vi "FTW-Actor-Initialized.vi"(0 "FTW Actor Instance":refnum<class "FTW-Actor-Instance.lvclass">, 5 "Initialized Response":string, 11 "error in":errorcluster) -> (4 "FTW Actor Instance out":refnum<class "FTW-Actor-Instance.lvclass">, 6 "Timed out?":bool, 15 "error out":errorcluster)   [LabVIEW 2013, in "FTW-Actor-Instance.lvclass"]
uses:
  FTW-Actor-Instance.lvclass
  FTW-Actor-FrameworkEvent.ctl
  FTW-Actor-Instance.lvclass/FTW-Actor-Instance.ctl
  time/FTW-Time-DisplayFormat-Timestamp.ctl
  socket/FTW-Socket-Type.ctl
  socket/FTW-Socket.lvclass
panel:
  # "Inputs"
  # "Outputs"
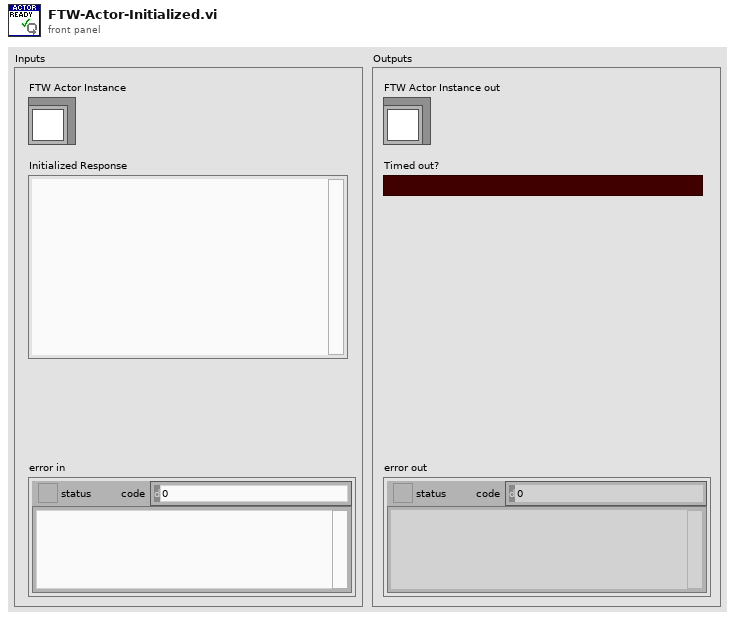
[diagram p1: front panel]
types:
  T1 = typedef "FTW-Actor-Instance.lvclass/FTW-Actor-FrameworkEvent.ctl" = enum16{"Instance Initializing", "Instance Initialized", "Instance Job", "Instance Handle Request", "Instance Shutting Down", "Instance Destroyed"}
  T2 = typedef "FTW-Time-DisplayFormat-Timestamp.ctl" = enum16{"YYYY-MM-DDT00:00:00.000Z (ISO-8601)", "YYYY-MM-DDT00-00-00Z (Simple ISO-8601)", "YYYY-MM-DD"}
  T3 = typedef "FTW-Socket.lvclass/FTW-Socket-Type.ctl" = enum32{"Server", "Client", "Publisher", "Subscriber", "Pipeline Producer", "Pipeline Consumer", "Surveyor", "Respondent", "Exclusive Pair", "Bus"}
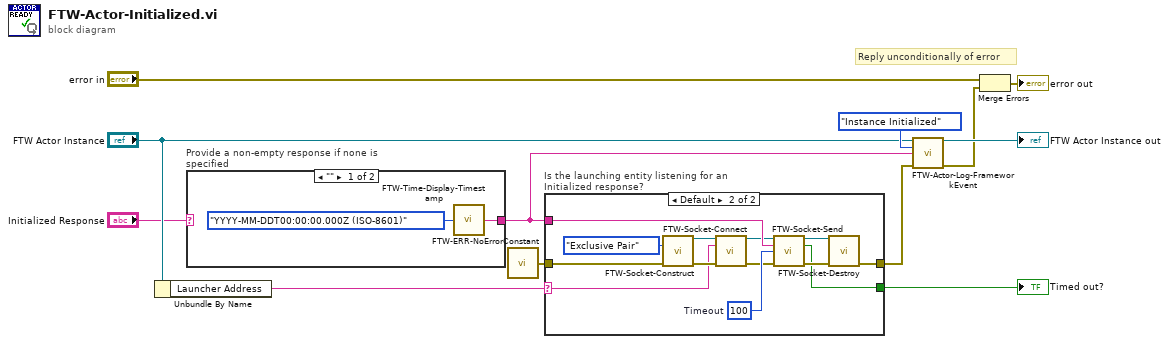
[diagram p0: block diagram]
diagram:
  # "Reply unconditionally of error"
  n1 = Unbundle By Name("FTW Actor Instance") -> ("Launcher Address"=w8:string)
  n2 = case "Provide a non-empty response if none is specified" shown="\"\"" "Initialized Response" {
    selector: "Initialized Response" -> [_ w15]
    tunnel: [w14 w15] -> w6
    frame "" {
      n3 = call "FTW-Time-Display-Timestamp.vi"("Format"=FTW-Time-DisplayFormat-Timestamp."YYYY-MM-DDT00:00:00.000Z (ISO-8601)") -> ("Formatted Timestamp"=w14:string)  [unwired: 3 in]
    }
    frame Default {
    }
  }
  n4 = call "FTW-ERR-NoErrorConstant.vi"() -> ("no error"=w5:errorcluster)
  n5 = case "Is the launching entity listening for an Initialized response?" shown="Default" w8 {
    selector: w8 -> [_ w21]
    tunnel: w6 -> [_ w28]
    tunnel: [w16 w26] -> w9
    tunnel: w5 -> [w16 w20]
    tunnel: [_ w18] -> w1
    frame "" {
    }
    frame Default {
      w25 = 100  # Timeout
      n6 = call "FTW-Socket-Construct.vi"("Socket Topology"=FTW-Socket-Type."Exclusive Pair" ("Socket Type"), "error in"=w20) -> ("FTW Socket"=w23:refnum<class "FTW-Socket.lvclass">, "error out"=w22:errorcluster)  [unwired: 12 in]
      n7 = call "FTW-Socket-Connect.vi"("FTW Socket"=w23, "Remote Address"=w21, "error in"=w22) -> ("FTW Socket out"=w19:refnum<class "FTW-Socket.lvclass">, "error out"=w17:errorcluster)  [unwired: 11 in]
      n8 = call "FTW-Socket-Send.vi"("FTW Socket"=w19, "Message"=w28, "Send Timeout"=w25, "error in"=w17) -> ("FTW Socket out"=w29:refnum<class "FTW-Socket.lvclass">, "Timed out?"=w18:bool, "error out"=w27:errorcluster)  [unwired: 9 in]
      n9 = call-dynamic "FTW-Socket-Destroy.vi"("FTW Socket"=w29, "error in"=w27) -> ("error out"=w26:errorcluster)  [unwired: 13 in]
    }
  }
  "Timed out?" <- w1
  n10 = call "FTW-Actor-Log-FrameworkEvent.vi"("FTW Actor Instance"="FTW Actor Instance", "Framework Event"=FTW-Actor-FrameworkEvent."Instance Initialized", "Event Data"=w6, "error in"=w9) -> ("FTW Actor Instance out"=→"FTW Actor Instance out":refnum<class "FTW-Actor-Instance.lvclass">, "error out"=w4:errorcluster)  [unwired: 10 in]
  n11 = Merge Errors("error in", w4) -> (→"error out":errorcluster)
